vi "Renishaw-XL80_SetMeasurementMode.vi"(8 "error in (no error)":errorcluster, 10 "MeasurementMode":i32(ring) items=["MEASUREMENT_INDETERMINATE", "MEASUREMENT_LINEAR_PLANE", "MEASUREMENT_LINEAR_RETRO", "MEASUREMENT_ANGULAR", "MEASUREMENT_STRAIGHTNESS_SHORT", "MEASUREMENT_STRAIGHTNESS_LONG", "MEASUREMENT_VELOCITY_RETRO"], 11 "Renishaw-XL80_EMU in":refnum<class "Renishaw-XL80_EMU.lvclass">) -> (0 "error out":errorcluster, 3 "Renishaw-XL80_EMU out":refnum<class "Renishaw-XL80_EMU.lvclass">)   [LabVIEW 2024, in "Renishaw-XL80_EMU.lvclass"]
doc: "MEASUREMENT_MODES\nThis enumerated type defines constants that specify the measurement mode.\n\nDefinition\n[v1_enum]typedef enum MEASUREMENT_MODES { MEASUREMENT_INDETERMINATE = 0, MEASUREMENT_LINEAR_PLANE = 1, MEASUREMENT_LINEAR_RETRO = 2, MEASUREMENT_ANGULAR = 3, MEASUREMENT_STRAIGHTNESS_SHORT = 4, MEASUREMENT_STRAIGHTNESS_LONG = 5} MEASUREMENT_MODES;\nComments\nThe v1_enum attribute indicates that the enumerated type will be transmitted as a 32-bit entity.\n\nMEASUREMENT_INDETERMINATE may be returned as part of the ML10 status. This would indicate that the ML10 is not responding. Attempting to use this value to set the measurement mode will fail. \nMEASUREMENT_LINEAR_PLANE indicates that the reading is treated as linear using a plane mirror. \nMEASUREMENT_LINEAR_RETRO indicates that the reading is treated as linear using a retro-reflector. \nMEASUREMENT_ANGULAR indicates that the reading is treated as angular. \nMEASUREMENT_STRAIGHTNESS_SHORT indicates that the reading is treated as straightness using short range optics. \nMEASUREMENT_STRAIGHTNESS_LONG indicates that the reading is treated as straightness using long range optics."
uses:
  Renishaw-XL80_EMU.lvclass
  Renishaw-XL80_EMU.lvclass/Renishaw-XL80_EMU.ctl
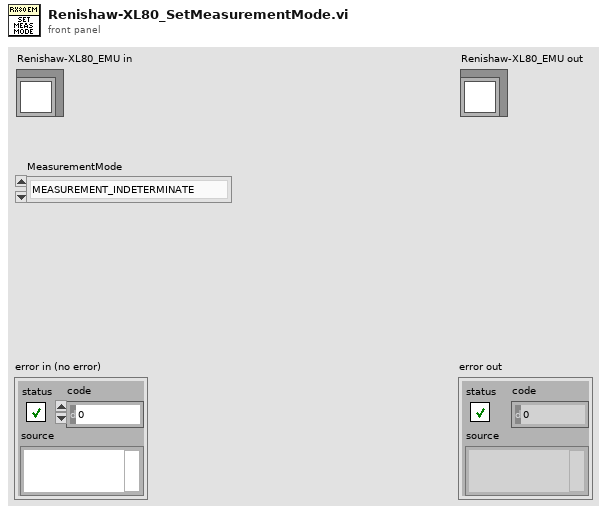
[diagram p1: front panel]
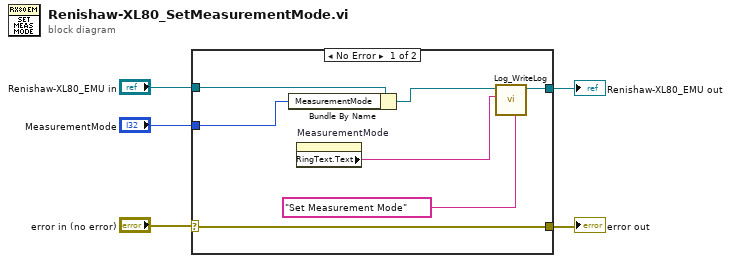
[diagram p0: block diagram]
diagram:
  n1 = case shown="No Error" "error in (no error)" {
    selector: "error in (no error)" -> [w12 w14]
    tunnel: [w12 w14] -> w4
    tunnel: [w8 w13] -> w3
    tunnel: "Renishaw-XL80_EMU in" -> [w11 w13]
    tunnel: "MeasurementMode" -> [w10 _]
    frame No Error {
      n2 = Bundle By Name(cluster=w11, "MeasurementMode"=w10) -> (w9:refnum<class "Renishaw-XL80_EMU.lvclass">)
      n3 = property on="MeasurementMode" class="Ring (strict)"() -> ("RingText.Text"=w6:string)  [unwired: 2 in, 2 out]
      n4 = call-dynamic "Log_WriteLog.vi"("Additional text"="Set Measurement Mode", "Command"=w6, "Log in"=w9) -> ("Log out"=w8:refnum<class "Renishaw-XL80_EMU.lvclass">)  [unwired: 7 in, 1 out]
    }
    frame Error {
    }
  }
  "error out" <- w4
  "Renishaw-XL80_EMU out" <- w3
